vi "connect_advertise.vi"(8 "错误输入（无错误）":errorcluster, 9 "type":string, 10 "topic":string, 11 "address":string="192.168.1.134") -> (0 "错误输出":errorcluster, 3 "连接ID输出":refnum<k5>)   [LabVIEW 2014]
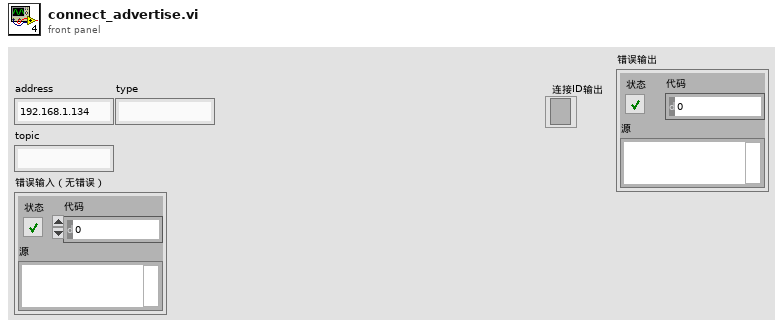
[diagram p1: front panel]
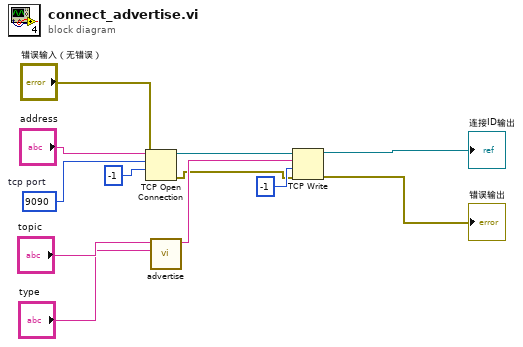
[diagram p0: block diagram]
diagram:
  w11 = u16 9090  # tcp port
  n1 = TCP Open Connection(address="address", remote port or service name=w11, timeout ms (60000)=-1 ("超时毫秒(60000)"), error in (no error)="错误输入（无错误）") -> (connection ID=w9:refnum<k5>, error out=w2:errorcluster)  [unwired: 1 in]
  n2 = call "advertise.vi"("type"="type", "topic"="topic") -> ("JSON string"=w5:string)  [unwired: 9 in]
  n3 = TCP Write(connection ID=w9, data in=w5, error in (no error)=w2, 9:-1 ("超时毫秒(25000)")) -> (connection ID out=→"连接ID输出":refnum<k5>, error out=→"错误输出":errorcluster)  [unwired: 1 out]
